vi "通用专用输入输出.vi"() -> ()   [LabVIEW 2011]
uses:
  <userlib>/LTDMC/LTDMC.lvlib
panel:
  in  "轴号":u16
  out "专用数字输入":u32
  out "专用输入信号":T1
  out "数字输入":u32
  out "数字输出回读":u32
  out "数字输出写入":u32
  in  "输出信号（鼠标点击）":T2
  out "输入信号":T3
  in  "退出":bool
  in  "卡号选择":u16(ring) items=["0"]
  out "init":bool
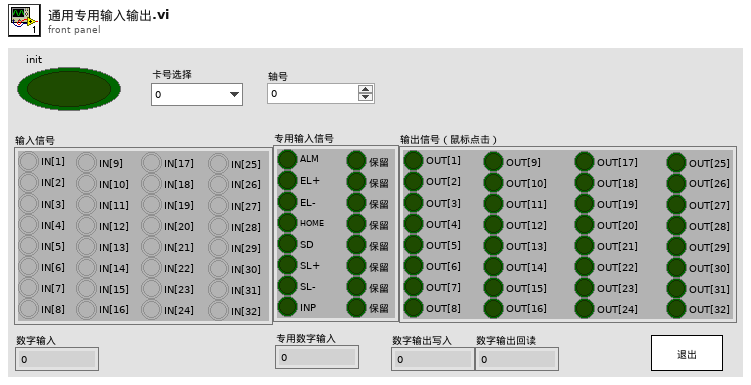
[diagram p1: front panel]
types:
  T1 = cluster{"ALM":bool, "EL+":bool, "EL-":bool, "HOME":bool, "SD":bool, "SL+":bool, "SL-":bool, "INP":bool, "保留":bool, "保留":bool, "保留":bool, "保留":bool, "保留":bool, "保留":bool, "保留":bool, "保留":bool}
  T2 = cluster{"OUT[1]":bool, "OUT[2]":bool, "OUT[3]":bool, "OUT[4]":bool, "OUT[5]":bool, "OUT[6]":bool, "OUT[7]":bool, "OUT[8]":bool, "OUT[9]":bool, "OUT[10]":bool, "OUT[11]":bool, "OUT[12]":bool, "OUT[13]":bool, "OUT[14]":bool, "OUT[15]":bool, "OUT[16]":bool, "OUT[17]":bool, "OUT[18]":bool, "OUT[19]":bool, "OUT[20]":bool, "OUT[21]":bool, "OUT[22]":bool, "OUT[23]":bool, "OUT[24]":bool, "OUT[25]":bool, "OUT[26]":bool, "OUT[27]":bool, "OUT[28]":bool, "OUT[29]":bool, "OUT[30]":bool, "OUT[31]":bool, "OUT[32]":bool}
  T3 = cluster{"IN[1]":bool, "IN[2]":bool, "IN[3]":bool, "IN[4]":bool, "IN[5]":bool, "IN[6]":bool, "IN[7]":bool, "IN[8]":bool, "IN[9]":bool, "IN[10]":bool, "IN[11]":bool, "IN[12]":bool, "IN[13]":bool, "IN[14]":bool, "IN[15]":bool, "IN[16]":bool, "IN[17]":bool, "IN[18]":bool, "IN[19]":bool, "IN[20]":bool, "IN[21]":bool, "IN[22]":bool, "IN[23]":bool, "IN[24]":bool, "IN[25]":bool, "IN[26]":bool, "IN[27]":bool, "IN[28]":bool, "IN[29]":bool, "IN[30]":bool, "IN[31]":bool, "IN[32]":bool}
  T4 = cluster{"Boolean array[0]":bool, "Boolean array[1]":bool, "Boolean array[2]":bool, "Boolean array[3]":bool, "Boolean array[4]":bool, "Boolean array[5]":bool, "Boolean array[6]":bool, "Boolean array[7]":bool, "Boolean array[8]":bool, "Boolean array[9]":bool, "Boolean array[10]":bool, "Boolean array[11]":bool, "Boolean array[12]":bool, "Boolean array[13]":bool, "Boolean array[14]":bool, "Boolean array[15]":bool, "Boolean array[16]":bool, "Boolean array[17]":bool, "Boolean array[18]":bool, "Boolean array[19]":bool, "Boolean array[20]":bool, "Boolean array[21]":bool, "Boolean array[22]":bool, "Boolean array[23]":bool, "Boolean array[24]":bool, "Boolean array[25]":bool, "Boolean array[26]":bool, "Boolean array[27]":bool, "Boolean array[28]":bool, "Boolean array[29]":bool, "Boolean array[30]":bool, "Boolean array[31]":bool}
  T5 = cluster{"Boolean array[0]":bool, "Boolean array[1]":bool, "Boolean array[2]":bool, "Boolean array[3]":bool, "Boolean array[4]":bool, "Boolean array[5]":bool, "Boolean array[6]":bool, "Boolean array[7]":bool, "Boolean array[8]":bool, "Boolean array[9]":bool, "Boolean array[10]":bool, "Boolean array[11]":bool, "Boolean array[12]":bool, "Boolean array[13]":bool, "Boolean array[14]":bool, "Boolean array[15]":bool}
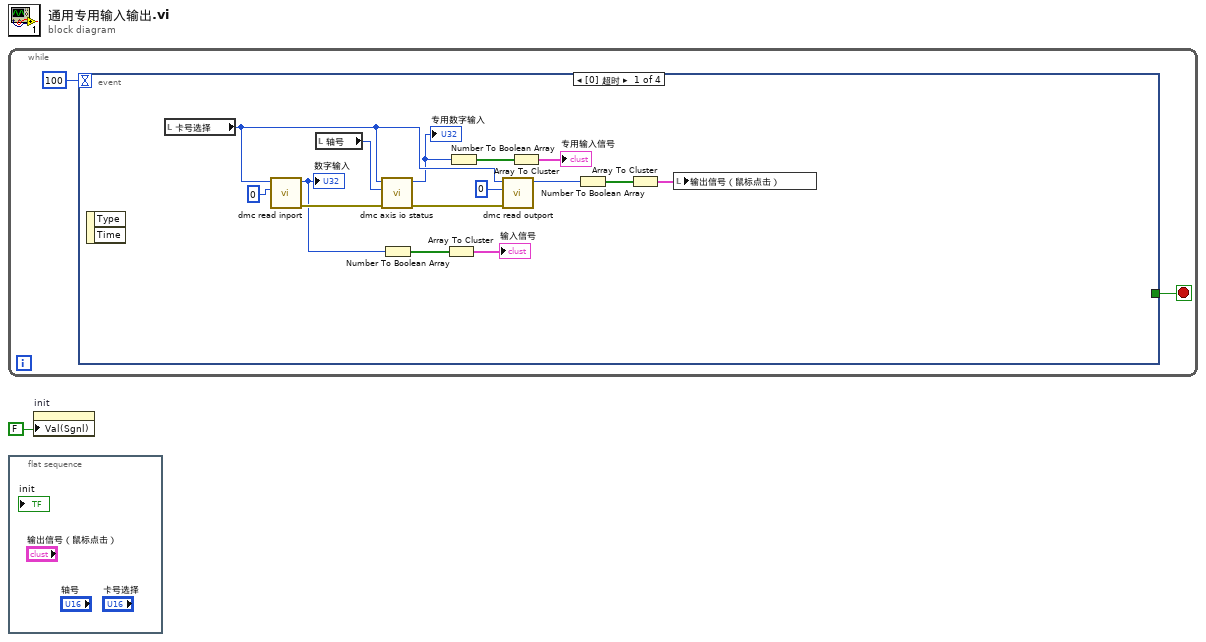
[diagram p0: block diagram]
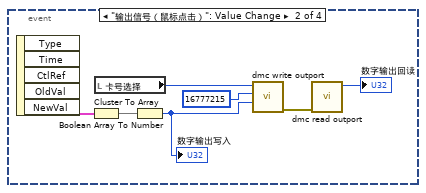
[diagram p2: hidden frame]
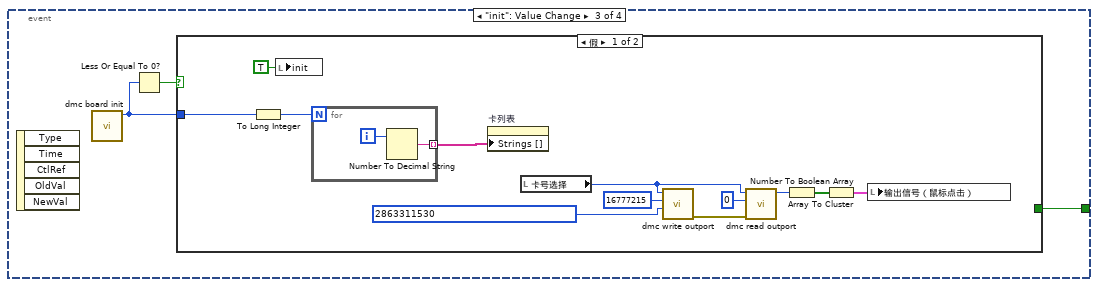
[diagram p3: hidden frame]
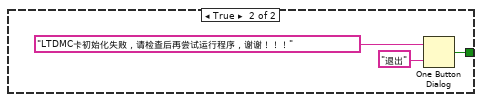
[diagram p4: hidden frame]
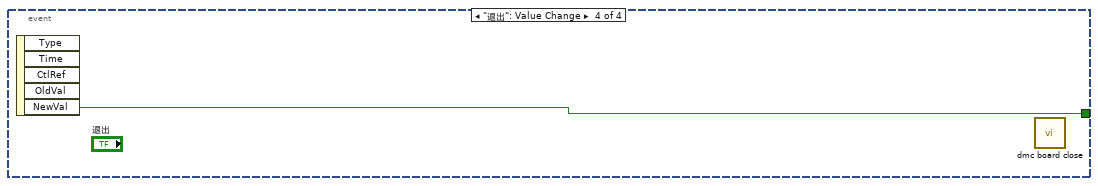
[diagram p5: hidden frame]
diagram:
  n1 = while {
    stop <- w3 stop-if-true
    n2 = event shown="[0] 超时" {
      selector: _ -> [_ _ _ _]
      dyn-events: _ -> [_ _ _ _]
      timeout: 100 -> [_ _ _ _]
      tunnel: [_ _ w27 w46] -> w3
      event Timeout {
        n3 = event-data() -> ()  [unwired: 1 in, 2 out]
        n4 = local read "卡号选择"() -> (w13:u16)
        n5 = call "dmc read inport.vi"("portno"=u16 0, "CardNo"=w13) -> ("error out"=w18:errorcluster, "function return"=w8:u32)  [unwired: 8 in]
        "数字输入" <- w8
        n6 = local read "轴号"() -> (w14:u16)
        n7 = call "dmc axis io status.vi"("error in (no error)"=w18, "axis"=w14, "CardNo"=w13) -> ("error out"=w17:errorcluster, "function return"=w6:u32)  [unwired: 7 in]
        "专用数字输入" <- w6
        n8 = Number To Boolean Array(number=w8) -> (Boolean array=w9:bool[])
        n9 = Array To Cluster(array=w9) -> (cluster=→"输入信号":T4)
        n10 = Number To Boolean Array(number=w6) -> (Boolean array=w4:bool[])
        n11 = call "dmc read outport.vi"("error in (no error)"=w17, "portno"=u16 0, "CardNo"=w13) -> ("function return"=w12:u32)  [unwired: 7 in, 1 out]
        n12 = Array To Cluster(array=w4) -> (cluster=→"专用输入信号":T5)
        n13 = Number To Boolean Array(number=w12) -> (Boolean array=w11:bool[])
        n14 = Array To Cluster(array=w11) -> (cluster=w10:T4)
        n15 = local write "输出信号（鼠标点击）"(w10) -> ()
      }
      event "输出信号（鼠标点击）": Value Change {
        n16 = event-data() -> ("NewVal"=w24:T2)  [unwired: 1 in, 4 out]
        n17 = Cluster To Array(cluster=w24) -> (array=w25:bool[])
        n18 = local read "卡号选择"() -> (w20:u16)
        n19 = Boolean Array To Number(Boolean array=w25) -> (number=w22:u32)
        "数字输出写入" <- w22
        n20 = call "dmc write outport.vi"("outport_val"=w22, "portno"=u32 16777215 ("IoMask"), "CardNo"=w20) -> ("error out"=w23:errorcluster)  [unwired: 7 in, 1 out]
        n21 = call "dmc read outport.vi"("error in (no error)"=w23) -> ("function return"=→"数字输出回读":u32)  [unwired: 9 in, 1 out]
      }
      event "init": Value Change {
        n22 = event-data() -> ()  [unwired: 1 in, 5 out]
        n23 = call "dmc board init.vi"() -> ("function return"=w26:i16)  [unwired: 10 in, 1 out]
        n24 = Less Or Equal To 0?(x=w26) -> (x <= 0?=w28:bool)
        n25 = case shown="假" w28 {
          tunnel: [_ w43] -> w27
          tunnel: w26 -> [w40 _]
          frame False {
            n26 = To Long Integer(number=w40) -> (32bit integer=w39:i32)
            n27 = local write "init"(TRUE ("init")) -> ()
            n28 = for {
              N: w39 -> [_]
              tunnel: [w41] -> w38 mode=indexing
              i -> [w42]
              n29 = Number To Decimal String(number=w42) -> (decimal integer string=w41:string)  [unwired: 1 in]
            }
            n30 = property on="卡列表" class="Ring (严格)"("Strings []"=w38) -> ()  [unwired: 2 in, 2 out]
            n31 = local read "卡号选择"() -> (w32:u16)
            n32 = call "dmc write outport.vi"("outport_val"=u32 2863311530 ("port_value"), "portno"=u32 16777215 ("IoMask"), "CardNo"=w32) -> ("error out"=w35:errorcluster)  [unwired: 7 in, 1 out]
            n33 = call "dmc read outport.vi"("error in (no error)"=w35, "portno"=u16 0, "CardNo"=w32) -> ("function return"=w30:u32)  [unwired: 7 in, 1 out]
            n34 = Number To Boolean Array(number=w30) -> (Boolean array=w29:bool[])
            n35 = Array To Cluster(array=w29) -> (cluster=w36:T4)
            n36 = local write "输出信号（鼠标点击）"(w36) -> ()
          }
          frame True {
            n37 = One Button Dialog(message="LTDMC卡初始化失败，请检查后再尝试运行程序，谢谢！！！" ("消息"), button name ("OK")="退出" ("按钮名称（“确定”）")) -> (true=w43:bool)
          }
        }
      }
      event "退出": Value Change {
        n38 = event-data() -> ("NewVal"=w46:bool)  [unwired: 1 in, 4 out]
        n39 = call "dmc board close.vi"() -> ()  [unwired: 10 in, 2 out]
      }
    }
  }
  n40 = flat-sequence {
    frame #0 {
    }
  }
  n41 = property on="init" class="Bool (严格)"("Val(Sgnl)"=FALSE ("值(信号)")) -> ()  [unwired: 2 in, 2 out]
